vi "Ctor.vi"(8 "error in (no error)":errorcluster, 11 "Element A in":refnum<class "Element B.lvclass">) -> (0 "error out":errorcluster, 3 "Element A out":refnum<class "Element B.lvclass">)   [LabVIEW 2014, in "Array Example.lvlib" / "Element B.lvclass"]
uses:
  Element B.lvclass
  Element Base/Element Base.lvclass
  Ref.ctl
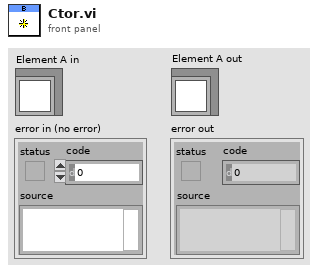
[diagram p1: front panel]
types:
  T1 = typedef "Array Example.lvlib/Element B.lvclass/Ref.ctl" = cluster{"Value":dbl}
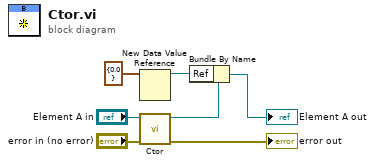
[diagram p0: block diagram]
diagram:
  n1 = New Data Value Reference(data value=T1 {"Value"=0.0} ("Ref")) -> (data value reference=w1:refnum<data-value>)  [unwired: 1 in, 1 out]
  n2 = call-parent "Ctor.vi"("error in (no error)"="error in (no error)", "ArrayPanel in"="Element A in") -> ("error out"=→"error out":errorcluster, "ArrayPanel out"=w5:refnum<class "Element B.lvclass">)  [unwired: 8 in]
  n3 = Bundle By Name(cluster=w5, "Ref"=w1) -> (→"Element A out":refnum<class "Element B.lvclass">)
